vi "Measurement Logic.vi"() -> ()   [LabVIEW 2021, in "Load Transient Response_PMIC.lvlib"]
uses:
  Load Transient Response_PMIC.lvlib
  Measurement Configuration.ctl
  Measurement Results.ctl
  <vilib>/MeasurementLink/MeasurementLink Measurement Server/Measure Call Context/Measure Call Context.lvclass
  <instrlib>/niDCPower/nidcpower.llb/niDCPower Sense.ctl
  <instrlib>/niDCPower/nidcpower.llb/niDCPower Source Mode.ctl
  <instrlib>/niDCPower/nidcpower.llb/niDCPower Wait For Event - Event.ctl
  <instrlib>/niDCPower/nidcpower.llb/niDCPower Output Function.ctl
  <instrlib>/niDCPower/nidcpower.llb/niDCPower Aperture Time Units.ctl
panel:
  out "measure call context out":refnum<class "Measure Call Context.lvclass">
  in  "measure call context in":refnum<class "Measure Call Context.lvclass">
  out "measurement results":T1
  in  "measurement configuration":T2={"Mode of operation"=enum."Perform measurement", "DUT setup time"=1.0, "Level dwell time"=0.001, "Nominal output voltage"=3.3, "Source resource name"="", "Source current limit"=25.0, "Source voltage level"=12.0, "Source voltage gain bandwidth"=2000.0, "Source voltage compensation frequency"=3530.0, "Source voltage pole-zero ratio"=2.0, "Load resource name"="", "Load voltage limit range"=6.0, "Load sample rate"=1800000.0, "Load current set point 1"=1.0, "Load current set point 2"=22.0, "Load current gain bandwidth"=14000.0, "Load current compensation frequency"=180000.0, "Load current pole-zero ratio"=0.3} {"Nominal output voltage" format="%#_6pV"; "Level dwell time" format="%#_6p"}
  out "error out":errorcluster
  in  "error in":errorcluster
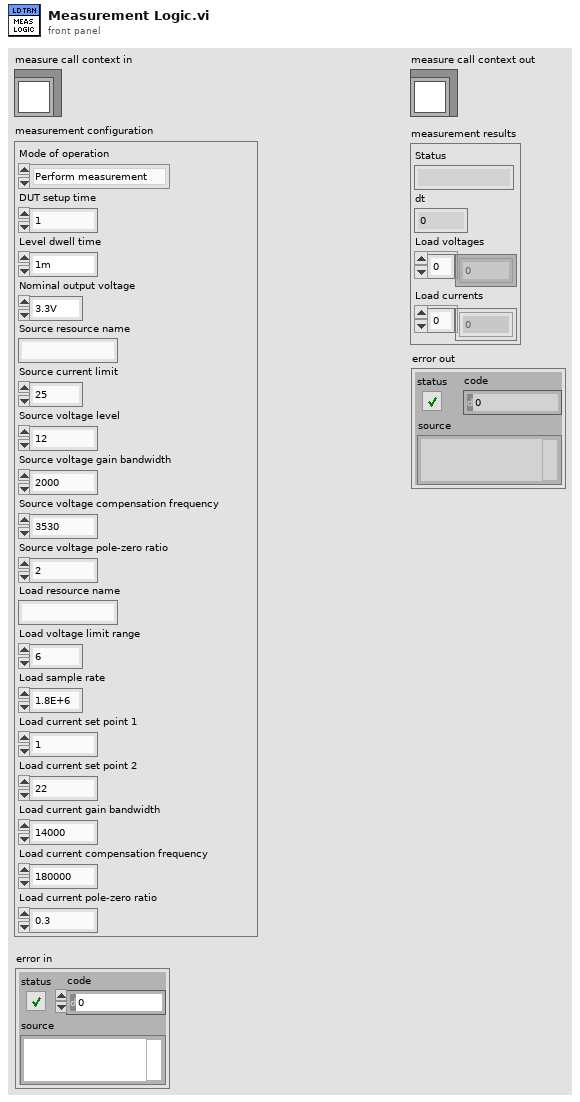
[diagram p1: front panel]
types:
  T1 = typedef "Load Transient Response_PMIC.lvlib/Measurement Results.ctl" = cluster{"Status":string, "dt":dbl, "Load voltages":dbl[], "Load currents":dbl[]}
  T2 = typedef "Load Transient Response_PMIC.lvlib/Measurement Configuration.ctl" = cluster{"Mode of operation":enum32{"Power on the DUT", "Perform measurement", "Power off the DUT"}, "DUT setup time":dbl, "Level dwell time":dbl, "Nominal output voltage":dbl, "Source resource name":string, "Source current limit":dbl, "Source voltage level":dbl, "Source voltage gain bandwidth":dbl, "Source voltage compensation frequency":dbl, "Source voltage pole-zero ratio":dbl, "Load resource name":string, "Load voltage limit range":dbl, "Load sample rate":dbl, "Load current set point 1":dbl, "Load current set point 2":dbl, "Load current gain bandwidth":dbl, "Load current compensation frequency":dbl, "Load current pole-zero ratio":dbl}
  T3 = cluster{"Source out":refnum<k15>, "Source channel name":string, "Load out":refnum<k15>, "Load channel name":string, "No of samples to fetch":i32, "Measurement Results":T1, "Source voltage level":dbl, "Source current limit":dbl}
  T4 = enum32{"Power on the DUT", "Perform measurement", "Power off the DUT"}
  T5 = typedef "niDCPower Wait For Event - Event.ctl" = i32
  T6 = typedef "niDCPower Source Mode.ctl" = i32
  T7 = typedef "niDCPower Sense.ctl" = i32
  T8 = typedef "niDCPower Output Function.ctl" = i32
  T9 = typedef "niDCPower Aperture Time Units.ctl" = i32
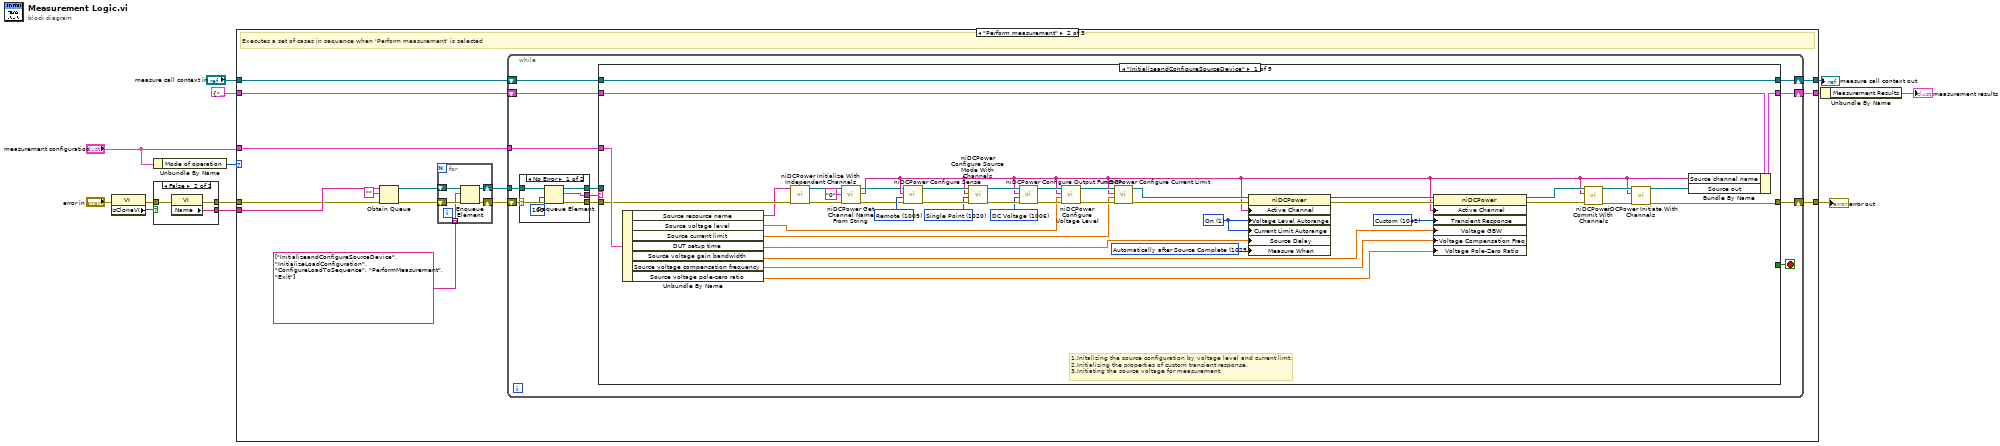
[diagram p0: block diagram]
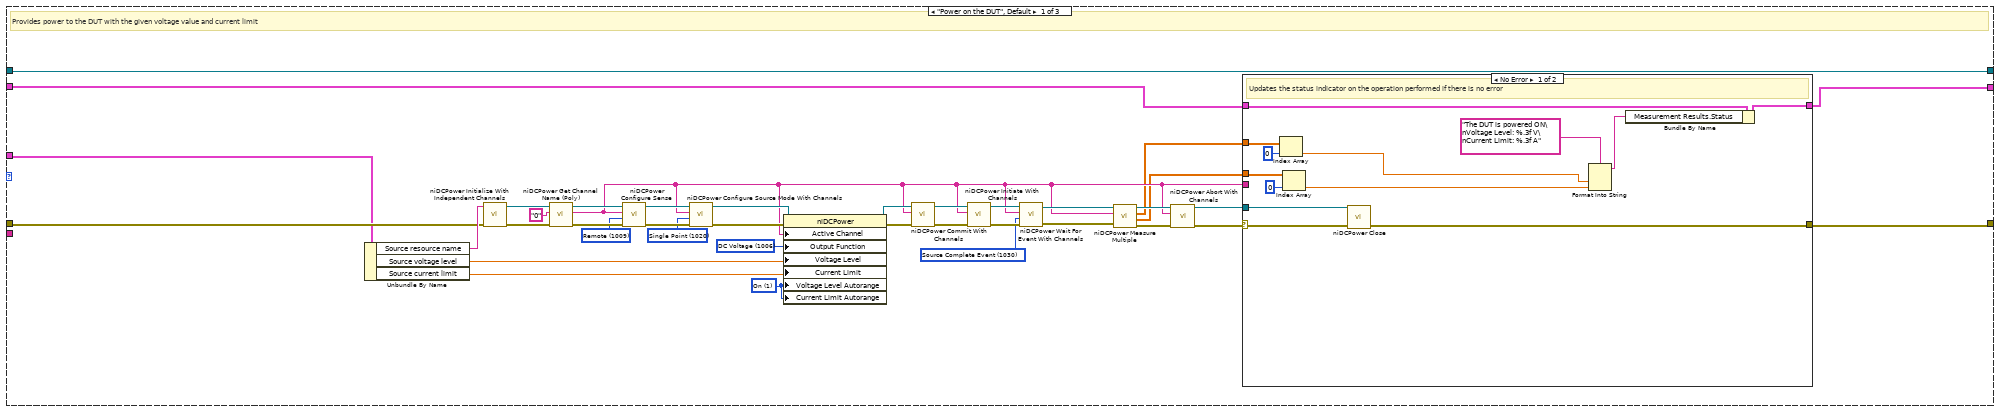
[diagram p2: hidden frame]
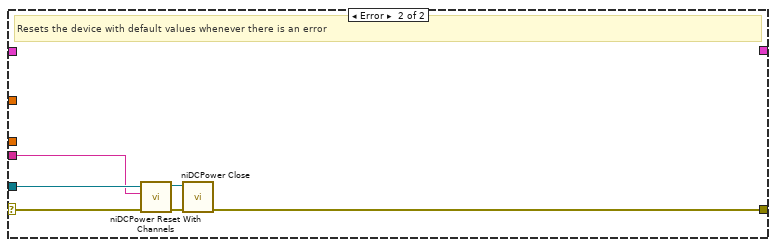
[diagram p3: hidden frame]
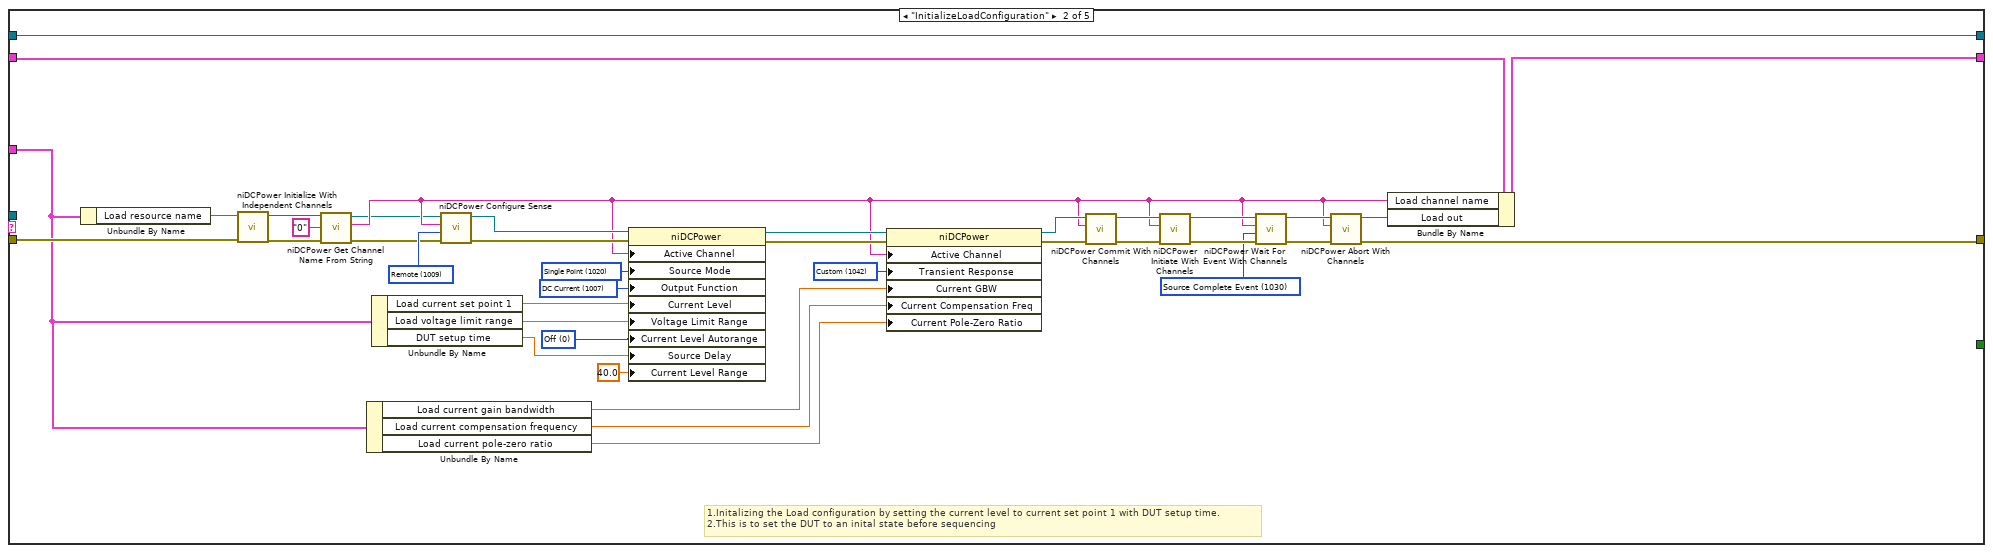
[diagram p4: hidden frame]
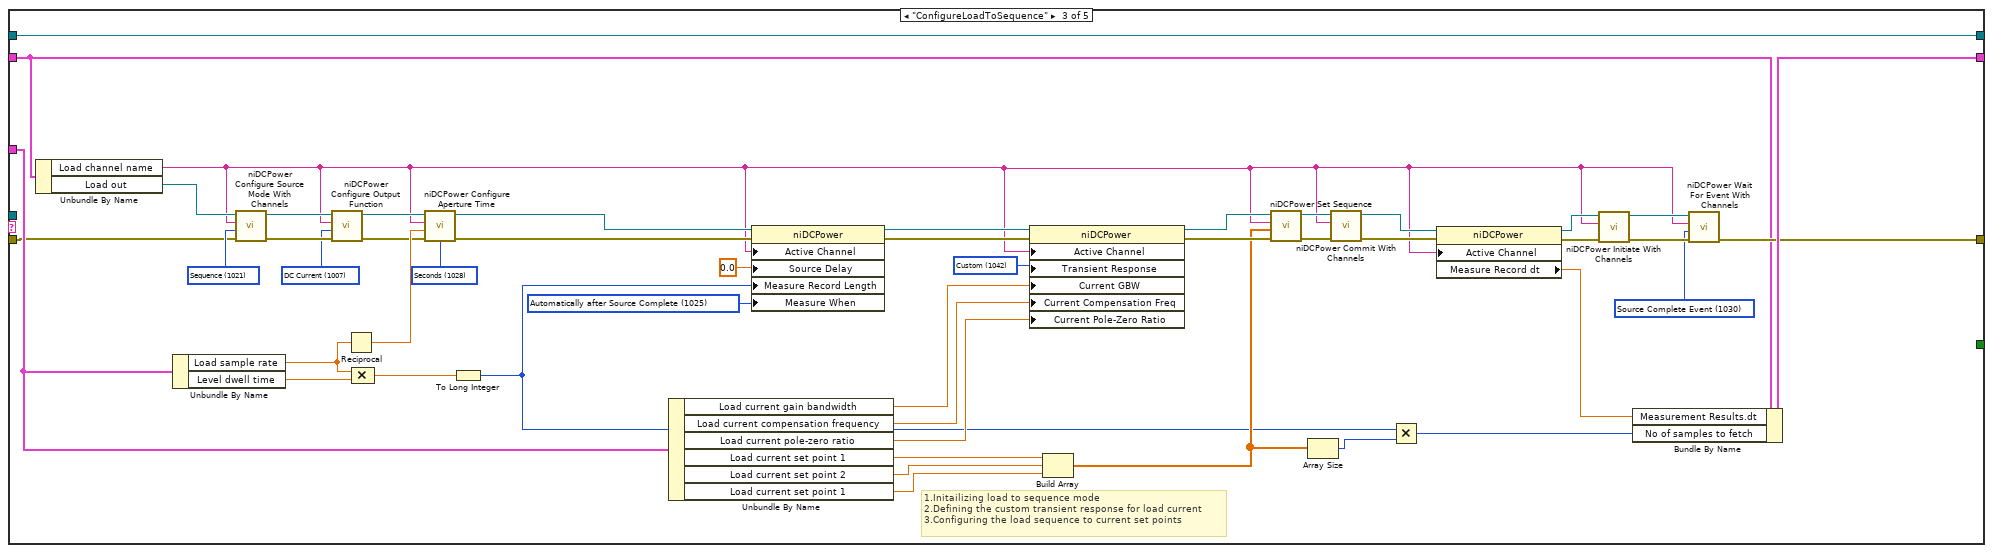
[diagram p5: hidden frame]
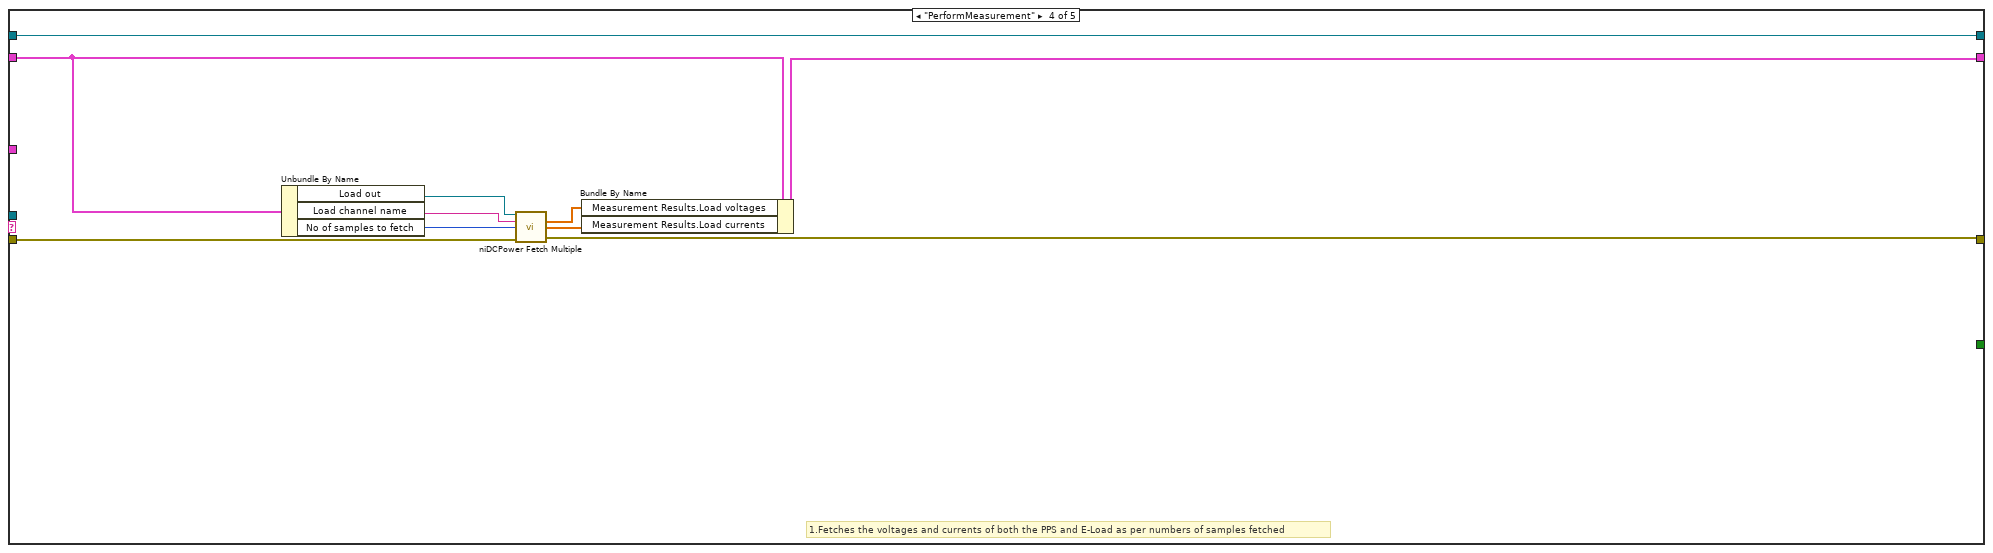
[diagram p6: hidden frame]
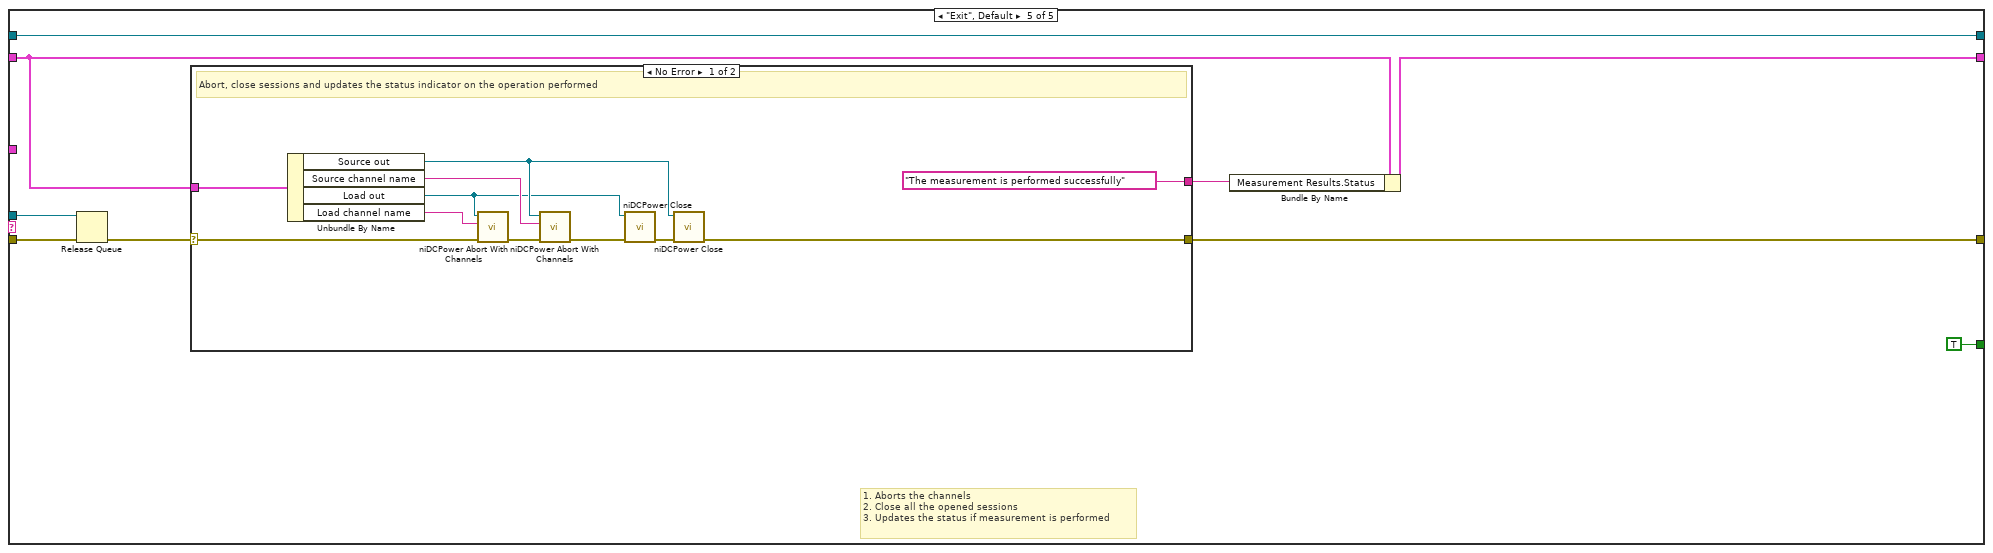
[diagram p7: hidden frame]
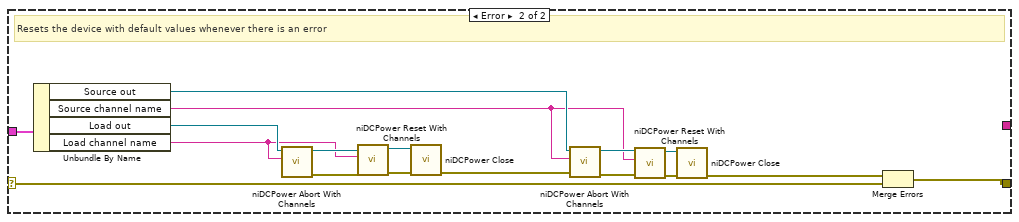
[diagram p8: hidden frame]
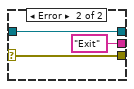
[diagram p9: hidden frame]
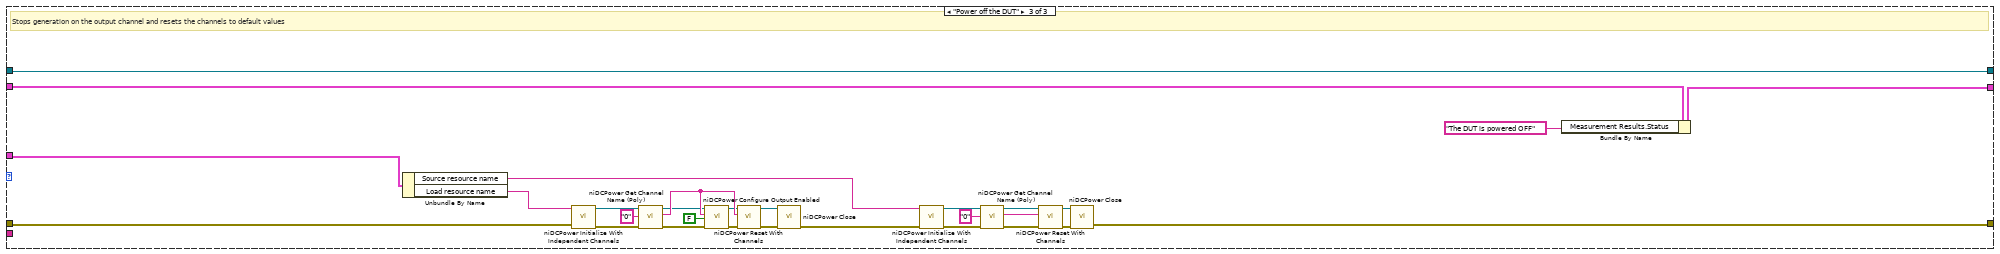
[diagram p10: hidden frame]
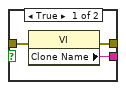
[diagram p11: hidden frame]
diagram:
  n1 = property class="VI"(error in="error in") -> (error out=w12:errorcluster, "IsCloneVI"=w13:bool)  [unwired: 1 in, 1 out]
  n2 = Unbundle By Name("measurement configuration") -> ("Mode of operation"=w2:T4)
  n3 = case shown="False" w13 {
    tunnel: [w16 w19] -> w4
    tunnel: [w15 w18] -> w1
    tunnel: w12 -> [w14 w17]
    frame True {
      n4 = property class="VI"(error in=w14) -> (error out=w16:errorcluster, "Clone Name"=w15:string)  [unwired: 1 in, 1 out]
    }
    frame False {
      n5 = property class="VI"(error in=w17) -> (error out=w19:errorcluster, "Name"=w18:string)  [unwired: 1 in, 1 out]
    }
  }
  n6 = case shown="\"Perform measurement\"" w2 {
    tunnel: T3 {"Source out"="", "Source channel name"="", "Load out"="", "Load channel name"="", "No of samples to fetch"=1, "Measurement Results"={"Status"="", "dt"=0.0, "Load voltages"=[], "Load currents"=[]}, "Source voltage level"=0.0, "Source current limit"=0.0} -> [w30 w89 w295]
    tunnel: "measure call context in" -> [w29 w88 w292]
    tunnel: [w21 w87 w296] -> w8
    tunnel: [w29 w86 w292] -> w6
    tunnel: [w20 w85 w293] -> w5
    tunnel: "measurement configuration" -> [w33 w84 w298]
    tunnel: w4 -> [w34 w77 w297]
    tunnel: w1 -> [_ w80 _]
    frame "Power on the DUT", Default {
      w38 = 1 items=["Off", "On"] ("Source:DC Voltage:Voltage Level Autorange")
      w37 = T5 1030 items=["Source Complete Event"=1030, "Measure Complete Event"=1031, "Sequence Iteration Complete Event"=1032, "Sequence Engine Done Event"=1033, "Pulse Complete Event"=1051, "Ready For Pulse Trigger Event"=1052] ("event")
      w36 = T6 1020 items=["Single Point"=1020, "Sequence"=1021] ("source mode")
      w39 = 1006 items=["DC Voltage"=1006, "DC Current"=1007, "Pulse Voltage"=1049, "Pulse Current"=1050] ("Source:Output Function")
      w40 = T7 1009 items=["Local"=1008, "Remote"=1009] ("sense")
      # "Provides power to the DUT with the given voltage value and current limit"
      n7 = Unbundle By Name(w33) -> ("Source resource name"=w54:string, "Source voltage level"=w55:dbl, "Source current limit"=w56:dbl)
      n8 = call <instrlib>:"niDCPower Initialize With Independent Channels.vi"("error in (no error)"=w34, "resource name"=w54) -> ("error out"=w52:errorcluster, "instrument handle out"=w51:refnum<k15>)  [unwired: 8 in]
      n9 = call-poly <instrlib>:"niDCPower Get Channel Name (Poly).vi"("index"="0", "instrument handle"=w51) -> ("name"=w26:string, "instrument handle out"=w53:refnum<k15>)  [unwired: 7 in, 1 out]
      n10 = call <instrlib>:"niDCPower Configure Sense.vi"("error in (no error)"=w52, "sense"=w40, "channel name"=w26, "instrument handle"=w53) -> ("error out"=w46:errorcluster, "instrument handle out"=w48:refnum<k15>)  [unwired: 6 in]
      n11 = call <instrlib>:"niDCPower Configure Source Mode With Channels.vi"("error in (no error)"=w46, "source mode"=w36, "channel name"=w26, "instrument handle"=w48) -> ("error out"=w45:errorcluster, "instrument handle out"=w47:refnum<k15>)  [unwired: 6 in]
      n12 = property class="niDCPower"(reference=w47, error in=w45, "Active Channel"=w26, "Output Function"=w39, "Voltage Level"=w55, "Current Limit"=w56, "Voltage Level Autorange"=w38, "Current Limit Autorange"=w38) -> (reference out=w44:refnum<k15>, error out=w43:errorcluster)
      n13 = call <instrlib>:"niDCPower Commit With Channels.vi"("error in (no error)"=w43, "channel name"=w26, "instrument handle"=w44) -> ("error out"=w41:errorcluster, "instrument handle out"=w42:refnum<k15>)  [unwired: 7 in]
      n14 = call <instrlib>:"niDCPower Initiate With Channels.vi"("error in (no error)"=w41, "channel name"=w26, "instrument handle"=w42) -> ("error out"=w50:errorcluster, "instrument handle out"=w49:refnum<k15>)  [unwired: 7 in]
      n15 = call <instrlib>:"niDCPower Wait For Event With Channels.vi"("error in (no error)"=w50, "event"=w37, "channel name"=w26, "instrument handle"=w49) -> ("error out"=w25:errorcluster, "instrument handle out"=w28:refnum<k15>)  [unwired: 6 in]
      n16 = call <instrlib>:"niDCPower Measure Multiple.vi"("error in (no error)"=w25, "channel name"=w26, "instrument handle"=w28) -> ("error out"=w24:errorcluster, "current measurements"=w22:dbl[], "voltage measurements"=w23:dbl[], "instrument handle out"=w27:refnum<k15>)  [unwired: 5 in]
      n17 = call <instrlib>:"niDCPower Abort With Channels.vi"("error in (no error)"=w24, "channel name"=w26, "instrument handle"=w27) -> ("error out"=w32:errorcluster, "instrument handle out"=w31:refnum<k15>)  [unwired: 7 in]
      n18 = case shown="No Error" w32 {
        selector: w32 -> [w68 w72]
        tunnel: [w67 w71] -> w21
        tunnel: w31 -> [w69 w73]
        tunnel: w26 -> [_ w70]
        tunnel: w30 -> [w66 _]
        tunnel: [w65 _] -> w20
        tunnel: w23 -> [w62 _]
        tunnel: w22 -> [w61 _]
        frame No Error {
          # "Updates the status indicator on the operation performed if there is no error"
          n19 = Index Array(array=w62, index=0) -> (element=w58:dbl)
          n20 = Index Array(array=w61, index=0) -> (element=w57:dbl)
          n21 = call <instrlib>:"niDCPower Close.vi"("error in (no error)"=w68, "instrument handle"=w69) -> ("error out"=w67:errorcluster)  [unwired: 9 out]
          n22 = Format Into String(format string="The DUT is powered ON\nVoltage Level: %.3f V\nCurrent Limit: %.3f A" ("message"), w58, w57) -> (resulting string=w63:string)  [unwired: 2 in, 1 out]
          n23 = Bundle By Name(cluster=w66, "Measurement Results.Status"=w63) -> (w65:T3)
        }
        frame Error {
          # "Resets the device with default values whenever there is an error"
          n24 = call <instrlib>:"niDCPower Reset With Channels.vi"("error in (no error)"=w72, "channel name"=w70, "instrument handle"=w73) -> ("error out"=w75:errorcluster, "instrument handle out"=w74:refnum<k15>)  [unwired: 7 in]
          n25 = call <instrlib>:"niDCPower Close.vi"("error in (no error)"=w75, "instrument handle"=w74) -> ("error out"=w71:errorcluster)  [unwired: 9 out]
        }
      }
    }
    frame "Perform measurement" {
      # "Executes a set of cases in sequence when 'Perform measurement' is selected"
      n26 = Obtain Queue(name (unnamed)=w80, element data type="", error in (no error)=w77) -> (queue out=w79:refnum<queue>, error out=w78:errorcluster)  [unwired: 2 in, 1 out]
      n27 = for {
        tunnel: string[] ["InitializeandConfigureSourceDevice", "InitializeLoadConfiguration", "ConfigureLoadToSequence", "PerformMeasurement", "Exit"] ("Step sequence") -> [w90] mode=indexing
        shift-right: [w93] -> w81
        shift-left: w79 -> [w92]
        shift-right: [w94] -> w82
        shift-left: w78 -> [w91]
        n28 = Enqueue Element(queue=w92, element=w90, error in (no error)=w91) -> (queue out=w93:refnum<queue>, error out=w94:errorcluster)  [unwired: 1 in, 1 out]
      }
      n29 = while {
        tunnel: w81 -> [w106]
        shift-right: [w99] -> w87
        shift-left: w82 -> [w105]
        tunnel: w84 -> [w101]
        shift-right: [w96] -> w86
        shift-left: w88 -> [w97]
        shift-right: [w95] -> w85
        shift-left: w89 -> [w98]
        stop <- w100 stop-if-true
        n30 = case shown="No Error" w105 {
          selector: w105 -> [w286 w290]
          tunnel: w106 -> [w288 w289]
          tunnel: [w287 "Exit" ("t")] -> w104
          tunnel: [w285 w290] -> w102
          tunnel: [w283 w289] -> w103
          frame No Error {
            n31 = Dequeue Element(queue=w288, timeout in ms (-1)=100, error in (no error)=w286) -> (queue out=w283:refnum<queue>, element=w287:string, error out=w285:errorcluster)  [unwired: 1 out]
          }
          frame Error {
          }
        }
        n32 = case shown="\"InitializeandConfigureSourceDevice\"" w104 {
          tunnel: w103 -> [_ _ _ _ w252]
          tunnel: w102 -> [w124 w171 w204 w243 w251]
          tunnel: w101 -> [w133 w169 w208 _ _]
          tunnel: [_ _ _ _ TRUE] -> w100
          tunnel: [w127 w160 w196 w241 w246] -> w99
          tunnel: w98 -> [w120 w164 w193 w244 w249]
          tunnel: w97 -> [w121 w161 w197 w245 w253]
          tunnel: [w121 w161 w197 w245 w253] -> w96
          tunnel: [w118 w162 w203 w242 w248] -> w95
          frame "InitializeandConfigureSourceDevice" {
            w132 = 1042 items=["Slow"=1041, "Normal"=1038, "Fast"=1039, "Custom"=1042] ("Source:Transient Response")
            w134 = T7 1009 items=["Local"=1008, "Remote"=1009] ("sense")
            w126 = 1025 items=["Automatically after Source Complete"=1025, "On Demand"=1026, "On Measure Trigger"=1027] ("Measurement:Advanced:Measure When")
            w135 = 1 items=["Off", "On"] ("Source:DC Voltage:Current Limit Autorange")
            w136 = T8 1006 items=["DC Voltage"=1006, "DC Current"=1007, "Pulse Voltage"=1049, "Pulse Current"=1050] ("output function")
            w137 = T6 1020 items=["Single Point"=1020, "Sequence"=1021] ("source mode")
            # "1.Initalizing the source configuration by voltage level and current limt.\n2.Initializing the properties of custom transient response.\n3.Initiating the source voltage for measurement."
            n33 = Unbundle By Name(w133) -> ("Source resource name"=w123:string, "Source voltage level"=w107:dbl, "Source current limit"=w108:dbl, "DUT setup time"=w109:dbl, "Source voltage gain bandwidth"=w125:dbl, "Source voltage compensation frequency"=w117:dbl, "Source voltage pole-zero ratio"=w122:dbl)
            n34 = call <instrlib>:"niDCPower Initialize With Independent Channels.vi"("error in (no error)"=w124, "resource name"=w123) -> ("error out"=w112:errorcluster, "instrument handle out"=w115:refnum<k15>)  [unwired: 8 in]
            n35 = call <instrlib>:"niDCPower Get Channel Name From String.vi"("error in (no error)"=w112, "index"="0", "instrument handle"=w115) -> ("error out"=w111:errorcluster, "name"=w114:string, "instrument handle out"=w113:refnum<k15>)  [unwired: 6 in]
            n36 = call <instrlib>:"niDCPower Configure Sense.vi"("error in (no error)"=w111, "sense"=w134, "channel name"=w114, "instrument handle"=w113) -> ("error out"=w147:errorcluster, "instrument handle out"=w148:refnum<k15>)  [unwired: 6 in]
            n37 = call <instrlib>:"niDCPower Configure Source Mode With Channels.vi"("error in (no error)"=w147, "source mode"=w137, "channel name"=w114, "instrument handle"=w148) -> ("error out"=w138:errorcluster, "instrument handle out"=w139:refnum<k15>)  [unwired: 6 in]
            n38 = call <instrlib>:"niDCPower Configure Output Function.vi"("error in (no error)"=w138, "output function"=w136, "channel name"=w114, "instrument handle"=w139) -> ("error out"=w141:errorcluster, "instrument handle out"=w142:refnum<k15>)  [unwired: 6 in]
            n39 = call <instrlib>:"niDCPower Configure Voltage Level.vi"("error in (no error)"=w141, "voltage level"=w107, "channel name"=w114, "instrument handle"=w142) -> ("error out"=w144:errorcluster, "instrument handle out"=w143:refnum<k15>)  [unwired: 6 in]
            n40 = call <instrlib>:"niDCPower Configure Current Limit.vi"("error in (no error)"=w144, "current limit"=w108, "channel name"=w114, "instrument handle"=w143) -> ("error out"=w140:errorcluster, "instrument handle out"=w116:refnum<k15>)  [unwired: 6 in]
            n41 = property class="niDCPower"(reference=w116, error in=w140, "Active Channel"=w114, "Voltage Level Autorange"=w135, "Current Limit Autorange"=w135, "Source Delay"=w109, "Measure When"=w126) -> (reference out=w131:refnum<k15>, error out=w129:errorcluster)
            n42 = property class="niDCPower"(reference=w131, error in=w129, "Active Channel"=w114, "Transient Response"=w132, "Voltage GBW"=w125, "Voltage Compensation Freq"=w117, "Voltage Pole-Zero Ratio"=w122) -> (reference out=w130:refnum<k15>, error out=w128:errorcluster)
            n43 = call <instrlib>:"niDCPower Commit With Channels.vi"("error in (no error)"=w128, "channel name"=w114, "instrument handle"=w130) -> ("error out"=w146:errorcluster, "instrument handle out"=w145:refnum<k15>)  [unwired: 7 in]
            n44 = call <instrlib>:"niDCPower Initiate With Channels.vi"("error in (no error)"=w146, "channel name"=w114, "instrument handle"=w145) -> ("error out"=w127:errorcluster, "instrument handle out"=w119:refnum<k15>)  [unwired: 7 in]
            n45 = Bundle By Name(cluster=w120, "Source channel name"=w114, "Source out"=w119) -> (w118:T3)
          }
          frame "InitializeLoadConfiguration" {
            w172 = 0 items=["Off", "On"] ("Source:DC Current:Current Level Autorange")
            w175 = 1042 items=["Slow"=1041, "Normal"=1038, "Fast"=1039, "Custom"=1042] ("Source:Transient Response")
            w182 = T5 1030 items=["Source Complete Event"=1030, "Measure Complete Event"=1031, "Sequence Iteration Complete Event"=1032, "Sequence Engine Done Event"=1033, "Pulse Complete Event"=1051, "Ready For Pulse Trigger Event"=1052] ("event")
            w185 = 1007 items=["DC Voltage"=1006, "DC Current"=1007, "Pulse Voltage"=1049, "Pulse Current"=1050] ("Source:Output Function")
            w186 = 1020 items=["Single Point"=1020, "Sequence"=1021] ("Source:Source Mode")
            w187 = T7 1009 items=["Local"=1008, "Remote"=1009] ("sense")
            # "1.Initalizing the Load configuration by setting the current level to current set point 1 with DUT setup time.\n2.This is to set the DUT to an inital state before sequencing"
            n46 = Unbundle By Name(w169) -> ("Load resource name"=w170:string)
            n47 = call <instrlib>:"niDCPower Initialize With Independent Channels.vi"("error in (no error)"=w171, "resource name"=w170) -> ("error out"=w151:errorcluster, "instrument handle out"=w155:refnum<k15>)  [unwired: 8 in]
            n48 = call <instrlib>:"niDCPower Get Channel Name From String.vi"("error in (no error)"=w151, "index"="0", "instrument handle"=w155) -> ("error out"=w152:errorcluster, "name"=w154:string, "instrument handle out"=w153:refnum<k15>)  [unwired: 6 in]
            n49 = Unbundle By Name(w169) -> ("Load current gain bandwidth"=w167:dbl, "Load current compensation frequency"=w166:dbl, "Load current pole-zero ratio"=w165:dbl)
            n50 = Unbundle By Name(w169) -> ("Load current set point 1"=w158:dbl, "Load voltage limit range"=w159:dbl, "DUT setup time"=w168:dbl)
            n51 = call <instrlib>:"niDCPower Configure Sense.vi"("error in (no error)"=w152, "sense"=w187, "channel name"=w154, "instrument handle"=w153) -> ("error out"=w178:errorcluster, "instrument handle out"=w179:refnum<k15>)  [unwired: 6 in]
            n52 = property class="niDCPower"(reference=w179, error in=w178, "Active Channel"=w154, "Source Mode"=w186, "Output Function"=w185, "Current Level"=w158, "Voltage Limit Range"=w159, "Current Level Autorange"=w172, "Source Delay"=w168, "Current Level Range"=40.0 ("Source:Advanced:Pulse Bias Delay")) -> (reference out=w174:refnum<k15>, error out=w173:errorcluster)
            n53 = property class="niDCPower"(reference=w174, error in=w173, "Active Channel"=w154, "Transient Response"=w175, "Current GBW"=w167, "Current Compensation Freq"=w166, "Current Pole-Zero Ratio"=w165) -> (reference out=w157:refnum<k15>, error out=w156:errorcluster)
            n54 = call <instrlib>:"niDCPower Commit With Channels.vi"("error in (no error)"=w156, "channel name"=w154, "instrument handle"=w157) -> ("error out"=w176:errorcluster, "instrument handle out"=w177:refnum<k15>)  [unwired: 7 in]
            n55 = call <instrlib>:"niDCPower Initiate With Channels.vi"("error in (no error)"=w176, "channel name"=w154, "instrument handle"=w177) -> ("error out"=w184:errorcluster, "instrument handle out"=w183:refnum<k15>)  [unwired: 7 in]
            n56 = call <instrlib>:"niDCPower Wait For Event With Channels.vi"("error in (no error)"=w184, "event"=w182, "channel name"=w154, "instrument handle"=w183) -> ("error out"=w181:errorcluster, "instrument handle out"=w180:refnum<k15>)  [unwired: 6 in]
            n57 = call <instrlib>:"niDCPower Abort With Channels.vi"("error in (no error)"=w181, "channel name"=w154, "instrument handle"=w180) -> ("error out"=w160:errorcluster, "instrument handle out"=w163:refnum<k15>)  [unwired: 7 in]
            n58 = Bundle By Name(cluster=w164, "Load channel name"=w154, "Load out"=w163) -> (w162:T3)
          }
          frame "ConfigureLoadToSequence" {
            w213 = 1042 items=["Slow"=1041, "Normal"=1038, "Fast"=1039, "Custom"=1042] ("Source:Transient Response")
            w191 = 1025 items=["Automatically after Source Complete"=1025, "On Demand"=1026, "On Measure Trigger"=1027] ("Measurement:Advanced:Measure When")
            w216 = T9 1028 items=["Seconds"=1028, "Powerline Cycles"=1029] ("aperture time units")
            w215 = T8 1007 items=["DC Voltage"=1006, "DC Current"=1007, "Pulse Voltage"=1049, "Pulse Current"=1050] ("output function")
            w217 = T5 1030 items=["Source Complete Event"=1030, "Measure Complete Event"=1031, "Sequence Iteration Complete Event"=1032, "Sequence Engine Done Event"=1033, "Pulse Complete Event"=1051, "Ready For Pulse Trigger Event"=1052] ("event")
            w218 = T6 1021 items=["Single Point"=1020, "Sequence"=1021] ("source mode")
            # "1.Initailizing load to sequence mode\n2.Defining the custom transient response for load current\n3.Configuring the load sequence to current set points"
            n59 = Unbundle By Name(w193) -> ("Load channel name"=w188:string, "Load out"=w210:refnum<k15>)
            n60 = Unbundle By Name(w208) -> ("Load sample rate"=w230:dbl, "Level dwell time"=w209:dbl)
            n61 = call <instrlib>:"niDCPower Configure Source Mode With Channels.vi"("error in (no error)"=w204, "source mode"=w218, "channel name"=w188, "instrument handle"=w210) -> ("error out"=w222:errorcluster, "instrument handle out"=w221:refnum<k15>)  [unwired: 6 in]
            n62 = call <instrlib>:"niDCPower Configure Output Function.vi"("error in (no error)"=w222, "output function"=w215, "channel name"=w188, "instrument handle"=w221) -> ("error out"=w224:errorcluster, "instrument handle out"=w223:refnum<k15>)  [unwired: 6 in]
            n63 = Reciprocal(x=w230) -> (1/x=w225:dbl)
            n64 = Compound Arithmetic op=MULTIPLY(w230, w209) -> (w227:dbl)
            n65 = call <instrlib>:"niDCPower Configure Aperture Time.vi"("aperture time units"=w216, "error in (no error)"=w224, "aperture time"=w225, "channel name"=w188, "instrument handle"=w223) -> ("error out"=w212:errorcluster, "instrument handle out"=w211:refnum<k15>)  [unwired: 5 in]
            n66 = To Long Integer(number=w227) -> (32bit integer=w192:i32)
            n67 = Unbundle By Name(w208) -> ("Load current gain bandwidth"=w207:dbl, "Load current compensation frequency"=w206:dbl, "Load current pole-zero ratio"=w205:dbl, "Load current set point 1"=w202:dbl, "Load current set point 2"=w201:dbl, "Load current set point 1"=w200:dbl)
            n68 = property class="niDCPower"(reference=w211, error in=w212, "Active Channel"=w188, "Source Delay"=0.0 ("Source:Advanced:Source Delay"), "Measure Record Length"=w192, "Measure When"=w191) -> (reference out=w232:refnum<k15>, error out=w233:errorcluster)
            n69 = property class="niDCPower"(reference=w232, error in=w233, "Active Channel"=w188, "Transient Response"=w213, "Current GBW"=w207, "Current Compensation Freq"=w206, "Current Pole-Zero Ratio"=w205) -> (reference out=w234:refnum<k15>, error out=w235:errorcluster)
            n70 = Build Array(w202, w201, w200) -> (w199:dbl[])
            n71 = call <instrlib>:"niDCPower Set Sequence.vi"("error in (no error)"=w235, "values"=w199, "channel name"=w188, "instrument handle"=w234) -> ("error out"=w189:errorcluster, "instrument handle out"=w190:refnum<k15>)  [unwired: 6 in]
            n72 = Array Size(array=w199) -> (size(s)=w198:i32)
            n73 = call <instrlib>:"niDCPower Commit With Channels.vi"("error in (no error)"=w189, "channel name"=w188, "instrument handle"=w190) -> ("error out"=w231:errorcluster, "instrument handle out"=w226:refnum<k15>)  [unwired: 7 in]
            n74 = Multiply(x=w192, y=w198) -> (x*y=w195:i32)
            n75 = property class="niDCPower"(reference=w226, error in=w231, "Active Channel"=w188) -> (reference out=w220:refnum<k15>, error out=w219:errorcluster, "Measure Record dt"=w194:dbl)
            n76 = call <instrlib>:"niDCPower Initiate With Channels.vi"("error in (no error)"=w219, "channel name"=w188, "instrument handle"=w220) -> ("error out"=w229:errorcluster, "instrument handle out"=w228:refnum<k15>)  [unwired: 7 in]
            n77 = Bundle By Name(cluster=w193, "Measurement Results.dt"=w194, "No of samples to fetch"=w195) -> (w203:T3)
            n78 = call <instrlib>:"niDCPower Wait For Event With Channels.vi"("error in (no error)"=w229, "event"=w217, "channel name"=w188, "instrument handle"=w228) -> ("error out"=w196:errorcluster)  [unwired: 6 in, 1 out]
          }
          frame "PerformMeasurement" {
            # "1.Fetches the voltages and currents of both the PPS and E-Load as per numbers of samples fetched"
            n79 = Unbundle By Name(w244) -> ("Load out"=w240:refnum<k15>, "Load channel name"=w239:string, "No of samples to fetch"=w237:i32)
            n80 = call <instrlib>:"niDCPower Fetch Multiple.vi"("instrument handle"=w240, "channel name"=w239, "count (1)"=w237, "error in (no error)"=w243) -> ("voltage measurements"=w238:dbl[], "current measurements"=w236:dbl[], "error out"=w241:errorcluster)  [unwired: 6 in, 3 out]
            n81 = Bundle By Name(cluster=w244, "Measurement Results.Load voltages"=w238, "Measurement Results.Load currents"=w236) -> (w242:T3)
          }
          frame "Exit", Default {
            # "1. Aborts the channels\n2. Close all the opened sessions\n3. Updates the status if measurement is performed"
            n82 = Release Queue(queue=w252, error in (no error)=w251) -> (error out=w250:errorcluster)  [unwired: 1 in, 2 out]
            n83 = case shown="No Error" w250 {
              selector: w250 -> [w258 w272]
              tunnel: w249 -> [w256 w273]
              tunnel: [w257 w271] -> w246
              tunnel: ["The measurement is performed successfully" ("message") _] -> w247
              frame No Error {
                # "Abort, close sessions and updates the status indicator on the operation performed"
                n84 = Unbundle By Name(w256) -> ("Source out"=w262:refnum<k15>, "Source channel name"=w264:string, "Load out"=w261:refnum<k15>, "Load channel name"=w263:string)
                n85 = call <instrlib>:"niDCPower Abort With Channels.vi"("error in (no error)"=w258, "channel name"=w263, "instrument handle"=w261) -> ("error out"=w265:errorcluster)  [unwired: 7 in, 1 out]
                n86 = call <instrlib>:"niDCPower Abort With Channels.vi"("error in (no error)"=w265, "channel name"=w264, "instrument handle"=w262) -> ("error out"=w260:errorcluster)  [unwired: 7 in, 1 out]
                n87 = call <instrlib>:"niDCPower Close.vi"("error in (no error)"=w260, "instrument handle"=w261) -> ("error out"=w259:errorcluster)  [unwired: 9 out]
                n88 = call <instrlib>:"niDCPower Close.vi"("error in (no error)"=w259, "instrument handle"=w262) -> ("error out"=w257:errorcluster)  [unwired: 9 out]
              }
              frame Error {
                # "Resets the device with default values whenever there is an error"
                n89 = Unbundle By Name(w273) -> ("Source out"=w267:refnum<k15>, "Source channel name"=w266:string, "Load out"=w269:refnum<k15>, "Load channel name"=w268:string)
                n90 = call <instrlib>:"niDCPower Abort With Channels.vi"("channel name"=w268, "instrument handle"=w269) -> ("error out"=w278:errorcluster, "instrument handle out"=w281:refnum<k15>)  [unwired: 8 in]
                n91 = call <instrlib>:"niDCPower Reset With Channels.vi"("error in (no error)"=w278, "channel name"=w268, "instrument handle"=w281) -> ("error out"=w277:errorcluster, "instrument handle out"=w276:refnum<k15>)  [unwired: 7 in]
                n92 = call <instrlib>:"niDCPower Close.vi"("error in (no error)"=w277, "instrument handle"=w276) -> ("error out"=w282:errorcluster)  [unwired: 9 out]
                n93 = call <instrlib>:"niDCPower Abort With Channels.vi"("error in (no error)"=w282, "channel name"=w266, "instrument handle"=w267) -> ("error out"=w280:errorcluster, "instrument handle out"=w279:refnum<k15>)  [unwired: 7 in]
                n94 = call <instrlib>:"niDCPower Reset With Channels.vi"("error in (no error)"=w280, "channel name"=w266, "instrument handle"=w279) -> ("error out"=w274:errorcluster, "instrument handle out"=w275:refnum<k15>)  [unwired: 7 in]
                n95 = call <instrlib>:"niDCPower Close.vi"("error in (no error)"=w274, "instrument handle"=w275) -> ("error out"=w270:errorcluster)  [unwired: 9 out]
                n96 = Merge Errors(w270, w272) -> (w271:errorcluster)
              }
            }
            n97 = Bundle By Name(cluster=w249, "Measurement Results.Status"=w247) -> (w248:T3)
          }
        }
      }
    }
    frame "Power off the DUT" {
      # "Stops generation on the output channel and resets the channels to default values"
      n98 = Unbundle By Name(w298) -> ("Source resource name"=w319:string, "Load resource name"=w316:string)
      n99 = call <instrlib>:"niDCPower Initialize With Independent Channels.vi"("error in (no error)"=w297, "resource name"=w316) -> ("error out"=w315:errorcluster, "instrument handle out"=w317:refnum<k15>)  [unwired: 8 in]
      n100 = call-poly <instrlib>:"niDCPower Get Channel Name (Poly).vi"("error in (no error)"=w315, "index"="0", "instrument handle"=w317) -> ("error out"=w308:errorcluster, "name"=w310:string, "instrument handle out"=w309:refnum<k15>)  [unwired: 6 in]
      n101 = call <instrlib>:"niDCPower Configure Output Enabled.vi"("error in (no error)"=w308, "output enabled"=FALSE, "channel name"=w310, "instrument handle"=w309) -> ("error out"=w302:errorcluster, "instrument handle out"=w303:refnum<k15>)  [unwired: 6 in]
      n102 = call <instrlib>:"niDCPower Reset With Channels.vi"("error in (no error)"=w302, "channel name"=w310, "instrument handle"=w303) -> ("error out"=w307:errorcluster, "instrument handle out"=w306:refnum<k15>)  [unwired: 7 in]
      n103 = call <instrlib>:"niDCPower Close.vi"("error in (no error)"=w307, "instrument handle"=w306) -> ("error out"=w312:errorcluster)  [unwired: 9 out]
      n104 = call <instrlib>:"niDCPower Initialize With Independent Channels.vi"("error in (no error)"=w312, "resource name"=w319) -> ("error out"=w318:errorcluster, "instrument handle out"=w320:refnum<k15>)  [unwired: 8 in]
      n105 = call-poly <instrlib>:"niDCPower Get Channel Name (Poly).vi"("error in (no error)"=w318, "index"="0", "instrument handle"=w320) -> ("error out"=w313:errorcluster, "name"=w314:string, "instrument handle out"=w311:refnum<k15>)  [unwired: 6 in]
      n106 = call <instrlib>:"niDCPower Reset With Channels.vi"("error in (no error)"=w313, "channel name"=w314, "instrument handle"=w311) -> ("error out"=w304:errorcluster, "instrument handle out"=w305:refnum<k15>)  [unwired: 7 in]
      n107 = call <instrlib>:"niDCPower Close.vi"("error in (no error)"=w304, "instrument handle"=w305) -> ("error out"=w296:errorcluster)  [unwired: 9 out]
      n108 = Bundle By Name(cluster=w295, "Measurement Results.Status"="The DUT is powered OFF" ("message")) -> (w293:T3)
    }
  }
  "error out" <- w8
  "measure call context out" <- w6
  n109 = Unbundle By Name(w5) -> ("Measurement Results"=→"measurement results":T1)
